vi "TaskScheduller.vi"(7 "TaskQuantity":dbl, 11 "TaskCounter":dbl) -> (2 "Boolean":bool, 3 "t":dbl)   [LabVIEW 2020]
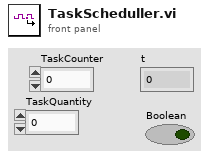
[diagram p1: front panel]
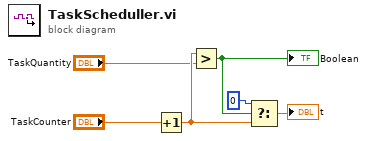
[diagram p0: block diagram]
diagram:
  n1 = Increment(x="TaskCounter") -> (x+1=w3:dbl)
  n2 = Greater?(x=w3, y="TaskQuantity") -> (0:w2:bool)
  "Boolean" <- w2
  n3 = Select(t=0, s=w2, f=w3) -> (s? t:f=→"t":dbl)
